vi "CRYProject Editor LIB.vi"(9 "sData":string, 11 "sAction":string) -> (2 "sData_Out":string)   [LabVIEW 2013]
uses:
  CRYProject Editor Global.vi
  CRYDocument/CRYReport Global.vi
  CRYSystem/Task Sequence/CRYProject Run Control Global.vi
  CRYMainGlobal.vi
  CRYSystem/Calibration/SubVI/CRYCal Global.vi
  CRYSystem/Program/CRYRef nums global.vi
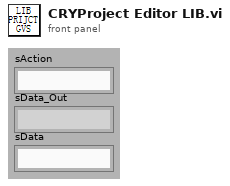
[diagram p1: front panel]
types:
  T1 = enum16{"New", "Open", "Close", "Close Data View Window Only", "Change", "Save", "Save for close"}
  T2 = enum16{"OK", "Yes", "YesNo", "YesNoCancel", "ReplaceAppend"}
  T3 = typedef "CRYTS.ctl" = cluster{"No.TS":u16, "TS File Path":path, "TS Name":string, "EditStepName":string, "Steps":T4[], "New State":bool, "Change State":bool, "Flattened CurveLib Data":string, "Document Data":string, "EditStepNo":u16, "Operator Start File":string, "Sequence Type":string, "Sequence Language":string}
  T4 = typedef "CRYStep.ctl" = cluster{"No.VI":i32, "Category":string, "StepName":string, "Seq setup flattened":string, "Comment":string, "Steps config.":bool[], "Jump config":i32[], "Start":dbl, "Increment":dbl, "Name":string, "Unit":string, "Y data":u16, "Y prefix":string, "Y dB ref":dbl, "Y unit":string, "Repeat State Array":cluster{"Start":dbl, "Increment":dbl, "Count":i32, "Num":i32}[]}
  T5 = enum16{"Left Button", "Center Button", "Right Button", "Window Close"}
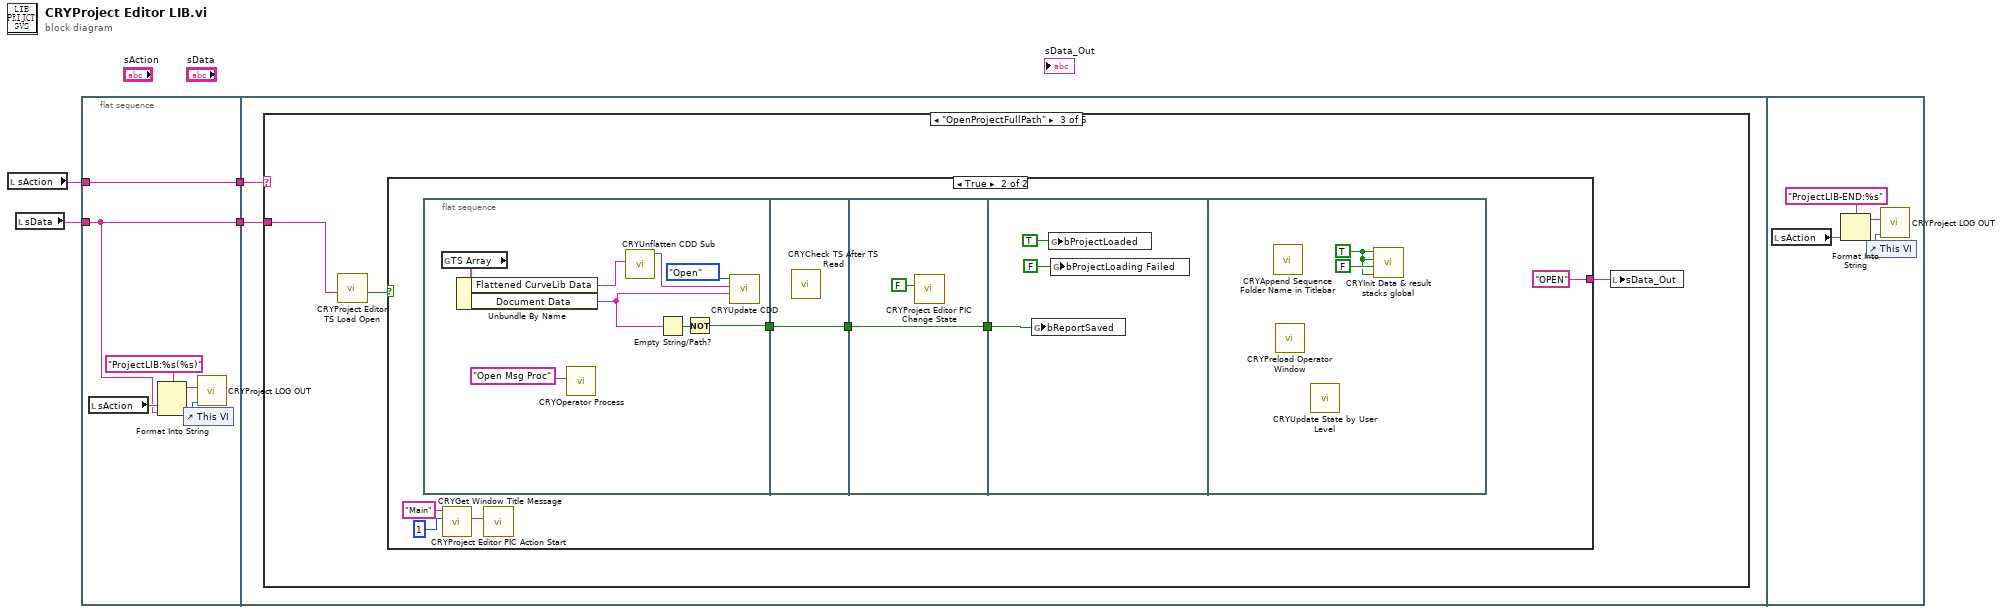
[diagram p0: block diagram]
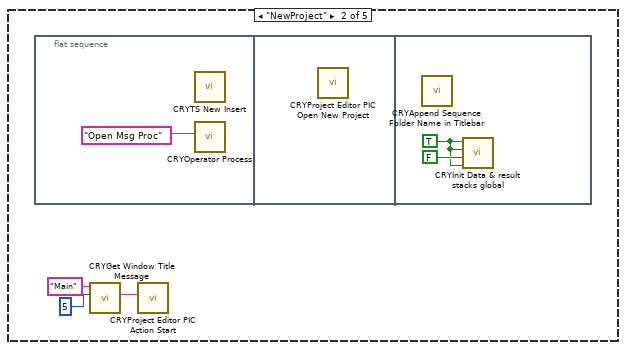
[diagram p3: hidden frame]
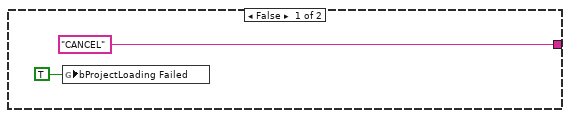
[diagram p4: hidden frame]
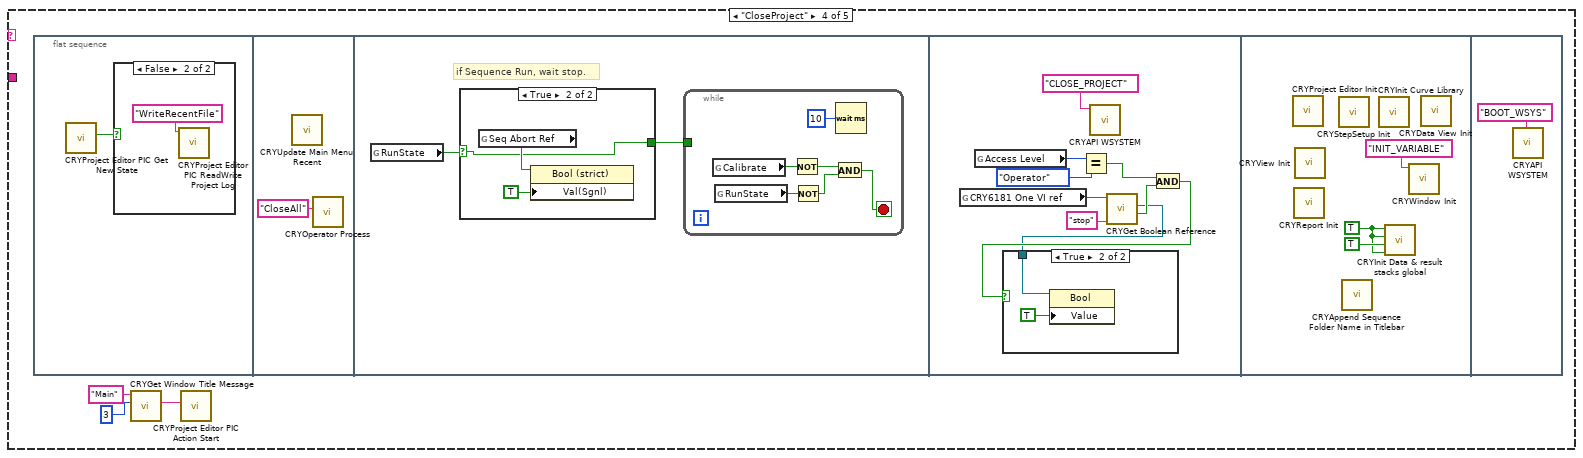
[diagram p5: hidden frame]
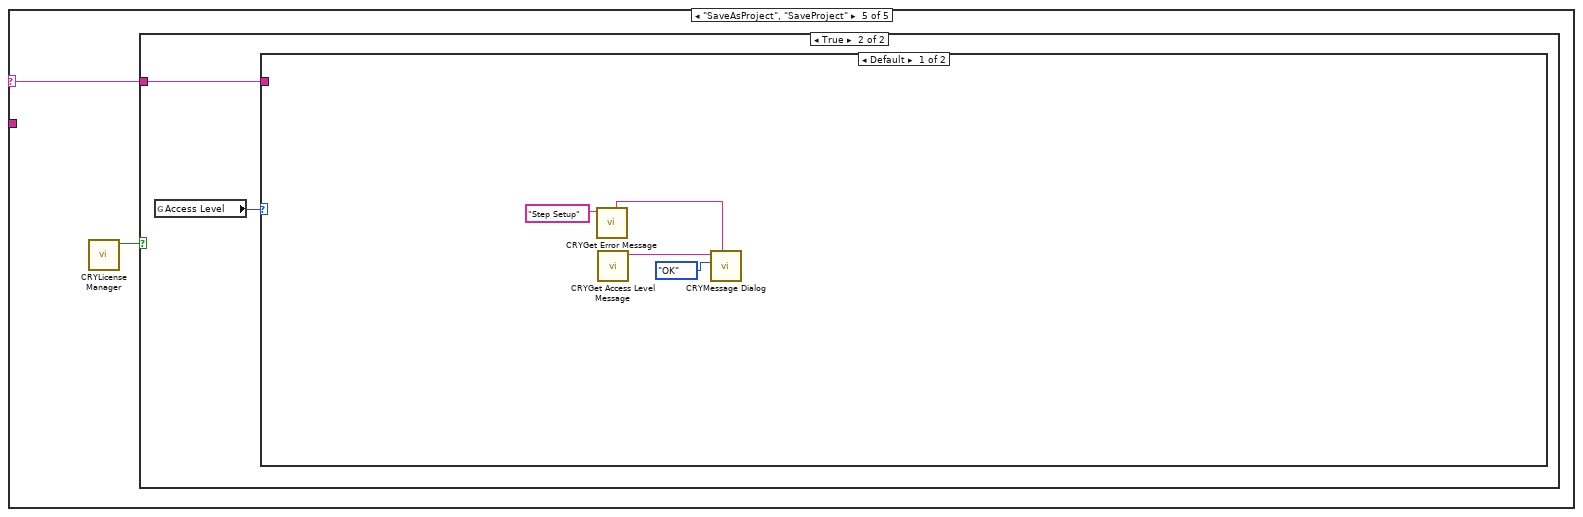
[diagram p9: hidden frame]
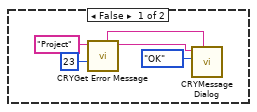
[diagram p10: hidden frame]
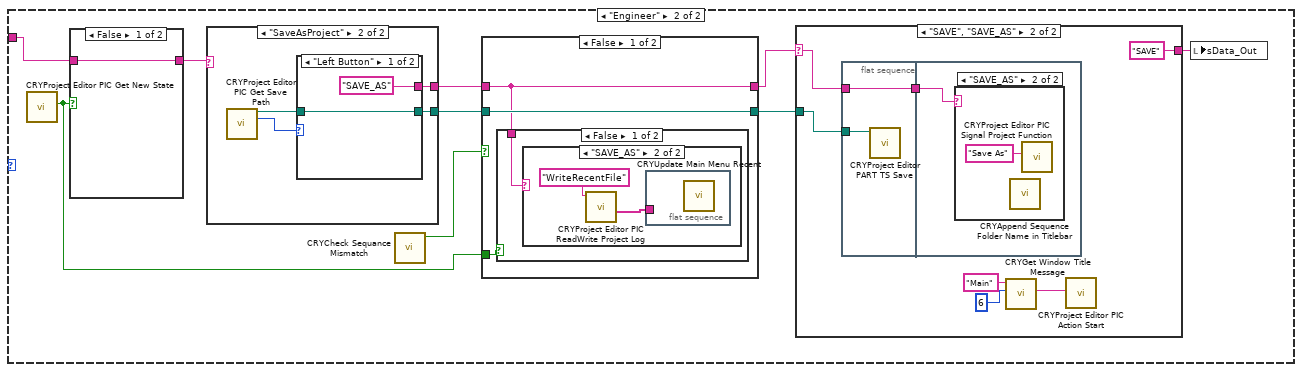
[diagram p11: hidden frame]
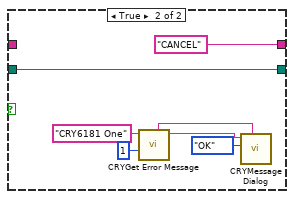
[diagram p14: hidden frame]
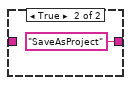
[diagram p15: hidden frame]
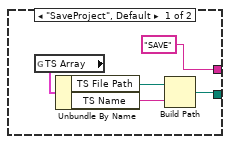
[diagram p18: hidden frame]
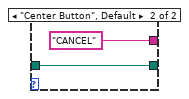
[diagram p19: hidden frame]
diagram:
  n1 = local read "sAction"() -> (w3:string)
  n2 = local read "sData"() -> (w1:string)
  n3 = flat-sequence {
    tunnel: w3 -> [w10]
    tunnel: [w10] -> w4
    tunnel: [w5] -> w2
    tunnel: w1 -> [w5]
    tunnel: w4 -> [w12]
    tunnel: w2 -> [w11]
    frame #0 {
      n4 = local read "sAction"() -> (w6:string)
      n5 = Format Into String(format string="ProjectLIB:%s(%s)", w6, w5) -> (resulting string=w8:string)  [unwired: 2 in, 1 out]
      n6 = control-ref of="This VI"() -> (w9:refnum<vi>)
      n7 = call "CRYProject LOG OUT.vi"("pVIRef"=w9, "sData"=w8) -> ()  [unwired: 10 in]
    }
    frame #1 {
      n8 = case shown="\"OpenProjectFullPath\"" w12 {
        selector: w12 -> [_ _ _ _ w81]
        tunnel: w11 -> [_ _ w20 _ _]
        frame "False", Default {
        }
        frame "NewProject" {
          n9 = flat-sequence {
            frame #0 {
              n10 = call "CRYTS New Insert.vi"() -> ()  [unwired: 1 in, 11 out]
              n11 = call "CRYOperator Process.vi"("sAction"="Open Msg Proc") -> ()  [unwired: 10 in, 1 out]
            }
            frame #1 {
              n12 = call "CRYProject Editor PIC Open New Project.vi"() -> ()  [unwired: 12 in]
            }
            frame #2 {
              w17 = TRUE ("Init?")
              n13 = call "CRYAppend Sequence Folder Name in Titlebar.vi"() -> ()  [unwired: 11 in]
              n14 = call "CRYInit Data & result stacks global.vi"("Set Value"=w17, "No Project Exist?"=FALSE ("New?"), "Pause Proc"=w17, "Init?"=w17) -> ()  [unwired: 8 in]
            }
          }
          n15 = call "CRYGet Window Title Message.vi"("No"=5, "Kind"="Main") -> ("Unicode String"=w13:string)  [unwired: 4 in, 5 out]
          n16 = call "CRYProject Editor PIC Action Start.vi"("sData"=w13) -> ()  [unwired: 11 in]
        }
        frame "OpenProjectFullPath" {
          n17 = call "CRYProject Editor TS Load Open.vi"("File Name"=w20) -> ("status"=w21:bool)  [unwired: 9 in]
          n18 = case shown="True" w21 {
            tunnel: ["CANCEL" "OPEN"] -> w19
            frame False {
              n19 = global write "CRYProject Editor Global.vi" "bProjectLoading Failed"(TRUE ("bProjectLoaded Failed")) -> ()
            }
            frame True {
              n20 = flat-sequence {
                tunnel: [w31] -> w29
                tunnel: [w39] -> w30
                tunnel: w29 -> [w39]
                tunnel: w30 -> [w41]
                tunnel: [w41] -> w24
                tunnel: w24 -> [w43]
                frame #0 {
                  n21 = global read "CRYProject Editor Global.vi" "TS Array"() -> (w37:T3)
                  n22 = Unbundle By Name(w37) -> ("Flattened CurveLib Data"=w36:string, "Document Data"=w33:string)
                  n23 = call "CRYOperator Process.vi"("sAction"="Open Msg Proc") -> ()  [unwired: 10 in, 1 out]
                  n24 = call "CRYUnflatten CDD Sub.vi"("Flatten Data In"=w36) -> ("Converted CDD"=w35:string)  [unwired: 9 in, 1 out]
                  n25 = Empty String/Path?(string/path=w33) -> (empty?=w32:bool)
                  n26 = Not(x=w32) -> (.not. x?=w31:bool)
                  n27 = call "CRYUpdate CDD.vi"("Document Data In"=w33, "Flatten Data In"=w35, "Signal"=T1."Open") -> ()  [unwired: 9 out]
                }
                frame #1 {
                  n28 = call "CRYCheck TS After TS Read.vi"() -> ()  [unwired: 1 out]
                }
                frame #2 {
                  n29 = call "CRYProject Editor PIC Change State.vi"("bChangeState"=FALSE) -> ()  [unwired: 11 in]
                }
                frame #3 {
                  n30 = global write "CRYReport Global.vi" "bReportSaved"(w43) -> ()
                  n31 = global write "CRYProject Editor Global.vi" "bProjectLoaded"(TRUE ("Project Exist?")) -> ()
                  n32 = global write "CRYProject Editor Global.vi" "bProjectLoading Failed"(FALSE ("bProjectLoaded Failed")) -> ()
                }
                frame #4 {
                  w45 = TRUE ("Init?")
                  n33 = call "CRYAppend Sequence Folder Name in Titlebar.vi"() -> ()  [unwired: 11 in]
                  n34 = call "CRYPreload Operator Window.vi"() -> ()  [unwired: 12 in]
                  n35 = call "CRYUpdate State by User Level.vi"() -> ()  [unwired: 12 in]
                  n36 = call "CRYInit Data & result stacks global.vi"("Set Value"=w45, "No Project Exist?"=FALSE ("New?"), "Pause Proc"=w45, "Init?"=w45) -> ()  [unwired: 8 in]
                }
              }
              n37 = call "CRYGet Window Title Message.vi"("No"=1, "Kind"="Main") -> ("Unicode String"=w26:string)  [unwired: 4 in, 5 out]
              n38 = call "CRYProject Editor PIC Action Start.vi"("sData"=w26) -> ()  [unwired: 11 in]
            }
          }
          n39 = local write "sData_Out"(w19) -> ()
        }
        frame "CloseProject" {
          n40 = flat-sequence {
            frame #0 {
              n41 = call "CRYProject Editor PIC Get New State.vi"() -> ("bNewState"=w50:bool)  [unwired: 11 in]
              n42 = case shown="False" w50 {
                frame True {
                }
                frame False {
                  n43 = call "CRYProject Editor PIC ReadWrite Project Log.vi"("sAction"="WriteRecentFile") -> ()  [unwired: 9 in, 2 out]
                }
              }
            }
            frame #1 {
              n44 = call "CRYUpdate Main Menu Recent.vi"() -> ()  [unwired: 12 in]
              n45 = call "CRYOperator Process.vi"("sAction"="CloseAll") -> ()  [unwired: 10 in, 1 out]
            }
            frame #2 {
              # "if Sequence Run, wait stop."
              n46 = global read "CRYProject Run Control Global.vi" "RunState"() -> (w54:bool)
              n47 = case shown="True" w54 {
                selector: w54 -> [w55 w56]
                tunnel: [w55 w56] -> w53
                frame False {
                }
                frame True {
                  n48 = global read "CRYMainGlobal.vi" "Seq Abort Ref"() -> (w58:refnum<vi>)
                  n49 = property class="Bool (strict)"(reference=w58, "Val(Sgnl)"=TRUE ("Value (Signaling)")) -> ()  [unwired: 1 in, 2 out]
                }
              }
              n50 = while {
                tunnel: w53 -> [_]
                stop <- w59 stop-if-true
                n51 = global read "CRYCal Global.vi" "Calibrate"() -> (w62:bool)
                n52 = global read "CRYProject Run Control Global.vi" "RunState"() -> (w64:bool)
                n53 = Not(x=w62) -> (.not. x?=w61:bool)
                n54 = Not(x=w64) -> (.not. x?=w60:bool)
                n55 = And(x=w61, y=w60) -> (x .and. y?=w59:bool)
                n56 = Wait (ms)(milliseconds to wait=u32 10) -> ()  [unwired: 1 out]
              }
            }
            frame #3 {
              n57 = global read "CRYRef nums global.vi" "CRY6181 One VI ref"() -> (w70:refnum<vi>)
              n58 = global read "CRYMainGlobal.vi" "Access Level"() -> (w72:enum16{"Engineer", "Technician", "Operator"})
              n59 = Equal?(x=w72, y=enum16{"Engineer", "Technician", "Operator"}."Operator") -> (x = y?=w69:bool)
              n60 = call "CRYAPI WSYSTEM.vi"("sAction"="CLOSE_PROJECT") -> ()  [unwired: 7 in, 4 out]
              n61 = call "CRYGet Boolean Reference.vi"("Label Name"="stop", "VI Refnum"=w70) -> ("Exist?"=w68:bool, "Boolean Ref"=w66:refnum<vi>)  [unwired: 8 out]
              n62 = And(x=w69, y=w68) -> (x .and. y?=w67:bool)
              n63 = case shown="True" w67 {
                tunnel: w66 -> [_ w75]
                frame False {
                }
                frame True {
                  n64 = property class="Bool"(reference=w75, "Value"=TRUE) -> ()  [unwired: 1 in, 2 out]
                }
              }
            }
            frame #4 {
              w76 = TRUE ("Init?")
              n65 = call "CRYProject Editor Init.vi"() -> ()  [unwired: 12 in]
              n66 = call "CRYReport Init.vi"() -> ()  [unwired: 12 in]
              n67 = call "CRYView Init.vi"() -> ()  [unwired: 12 in]
              n68 = call "CRYStepSetup Init.vi"() -> ()  [unwired: 12 in]
              n69 = call "CRYAppend Sequence Folder Name in Titlebar.vi"() -> ()  [unwired: 11 in]
              n70 = call "CRYInit Curve Library.vi"() -> ()  [unwired: 1 in]
              n71 = call "CRYInit Data & result stacks global.vi"("Set Value"=w76, "No Project Exist?"=TRUE ("New?"), "Pause Proc"=w76, "Init?"=w76) -> ()  [unwired: 8 in]
              n72 = call "CRYWindow Init.vi"("sAction"="INIT_VARIABLE") -> ()  [unwired: 11 in]
              n73 = call "CRYData View Init.vi"() -> ()  [unwired: 12 in]
            }
            frame #5 {
              n74 = call "CRYAPI WSYSTEM.vi"("sAction"="BOOT_WSYS") -> ()  [unwired: 7 in, 4 out]
            }
          }
          n75 = call "CRYGet Window Title Message.vi"("No"=3, "Kind"="Main") -> ("Unicode String"=w47:string)  [unwired: 4 in, 5 out]
          n76 = call "CRYProject Editor PIC Action Start.vi"("sData"=w47) -> ()  [unwired: 11 in]
        }
        frame "SaveAsProject", "SaveProject" {
          n77 = call "CRYLicense Manager.vi"() -> ("Test Result"=w80:bool)  [unwired: 10 in, 1 out]
          n78 = case shown="True" w80 {
            tunnel: w81 -> [_ w88]
            frame False {
              n79 = call "CRYGet Error Message.vi"("Error No"=23, "Kind"="Project") -> ("Message"=w82:string, "Window Title"=w86:string)  [unwired: 4 in, 4 out]
              n80 = call "CRYMessage Dialog.vi"("Window Title"=w86, "YesNoCancel"=T2."OK", "Message Content"=w82) -> ()  [unwired: 7 in, 2 out]
            }
            frame True {
              n81 = global read "CRYMainGlobal.vi" "Access Level"() -> (w87:enum16{"Engineer", "Technician", "Operator"})
              n82 = case shown="Default" w87 {
                tunnel: w88 -> [_ w101]
                frame Default {
                  n83 = call "CRYGet Error Message.vi"("Kind"="Step Setup") -> ("Window Title"=w90:string)  [unwired: 5 in, 5 out]
                  n84 = call "CRYGet Access Level Message.vi"() -> ("Multibyte string"=w92:string)  [unwired: 11 in]
                  n85 = call "CRYMessage Dialog.vi"("Window Title"=w90, "YesNoCancel"=T2."OK", "Message Content"=w92) -> ()  [unwired: 7 in, 2 out]
                }
                frame "Engineer" {
                  n86 = call "CRYProject Editor PIC Get New State.vi"() -> ("bNewState"=w93:bool)  [unwired: 11 in]
                  n87 = case shown="False" w93 {
                    tunnel: w101 -> [w115 _]
                    tunnel: [w115 "SaveAsProject"] -> w100
                    frame False {
                    }
                    frame True {
                    }
                  }
                  n88 = case shown="\"SaveAsProject\"" w100 {
                    tunnel: ["SAVE" w135] -> w98
                    tunnel: [w130 w134] -> w97
                    frame "SaveProject", Default {
                      n89 = global read "CRYProject Editor Global.vi" "TS Array"() -> (w133:T3)
                      n90 = Unbundle By Name(w133) -> ("TS File Path"=w131:path, "TS Name"=w129:string)
                      n91 = Build Path(base path=w131, name or relative path=w129) -> (appended path=w130:path)
                    }
                    frame "SaveAsProject" {
                      n92 = call "CRYProject Editor PIC Get Save Path.vi"() -> ("Path"=w136:path, "Which Button?"=w137:T5)  [unwired: 13 in, 1 out]
                      n93 = case shown="\"Left Button\"" w137 {
                        tunnel: w136 -> [w139 w140]
                        tunnel: ["SAVE_AS" "CANCEL"] -> w135
                        tunnel: [w139 w140] -> w134
                        frame "Left Button" {
                        }
                        frame "Center Button", Default {
                        }
                      }
                    }
                  }
                  n94 = call "CRYCheck Sequance Mismatch.vi"() -> ("Mismatch"=w94:bool)  [unwired: 10 in, 1 out]
                  n95 = case shown="False" w94 {
                    tunnel: [w103 "CANCEL"] -> w96
                    tunnel: w98 -> [w103 _]
                    tunnel: w97 -> [w104 w108]
                    tunnel: [w104 w108] -> w95
                    tunnel: w93 -> [w102 _]
                    frame False {
                      n96 = case shown="False" w102 {
                        tunnel: w103 -> [w105 _]
                        frame False {
                          n97 = case shown="\"SAVE_AS\"" w105 {
                            frame Default {
                            }
                            frame "SAVE_AS" {
                              n98 = call "CRYProject Editor PIC ReadWrite Project Log.vi"("sAction"="WriteRecentFile") -> ("sDataList_Out"=w106:string[])  [unwired: 9 in, 1 out]
                              n99 = flat-sequence {
                                tunnel: w106 -> [_]
                                frame #0 {
                                n100 = call "CRYUpdate Main Menu Recent.vi"() -> ()  [unwired: 12 in]
                                }
                              }
                            }
                          }
                        }
                        frame True {
                        }
                      }
                    }
                    frame True {
                      n101 = call "CRYGet Error Message.vi"("Error No"=1, "Kind"="CRY6181 One") -> ("Message"=w112:string, "Window Title"=w111:string)  [unwired: 4 in, 4 out]
                      n102 = call "CRYMessage Dialog.vi"("Window Title"=w111, "YesNoCancel"=T2."OK", "Message Content"=w112) -> ()  [unwired: 7 in, 2 out]
                    }
                  }
                  n103 = case shown="\"SAVE\", \"SAVE_AS\"" w96 {
                    selector: w96 -> [w117 w121]
                    tunnel: w95 -> [_ w124]
                    tunnel: [w117 "SAVE"] -> w99
                    frame "CANCEL", Default {
                    }
                    frame "SAVE", "SAVE_AS" {
                      n104 = flat-sequence {
                        tunnel: [w125] -> w122
                        tunnel: w121 -> [w125]
                        tunnel: w124 -> [w126]
                        tunnel: w122 -> [w127]
                        frame #0 {
                          n105 = call "CRYProject Editor PART TS Save.vi"("pSaveName"=w126) -> ()  [unwired: 11 in]
                        }
                        frame #1 {
                          n106 = case shown="\"SAVE_AS\"" w127 {
                            frame "False", Default {
                            }
                            frame "SAVE_AS" {
                              n107 = call "CRYAppend Sequence Folder Name in Titlebar.vi"() -> ()  [unwired: 11 in]
                              n108 = call "CRYProject Editor PIC Signal Project Function.vi"("sData"="Save As") -> ()  [unwired: 11 in]
                            }
                          }
                        }
                      }
                      n109 = call "CRYGet Window Title Message.vi"("No"=6, "Kind"="Main") -> ("Unicode String"=w118:string)  [unwired: 4 in, 5 out]
                      n110 = call "CRYProject Editor PIC Action Start.vi"("sData"=w118) -> ()  [unwired: 11 in]
                    }
                  }
                  n111 = local write "sData_Out"(w99) -> ()
                }
              }
            }
          }
        }
      }
    }
    frame #2 {
      n112 = local read "sAction"() -> (w142:string)
      n113 = Format Into String(format string="ProjectLIB-END:%s", w142) -> (resulting string=w144:string)  [unwired: 2 in, 1 out]
      n114 = control-ref of="This VI"() -> (w145:refnum<vi>)
      n115 = call "CRYProject LOG OUT.vi"("pVIRef"=w145, "sData"=w144) -> ()  [unwired: 10 in]
    }
  }
